vi "OutputBitAssignments.vi"(0 "System":u16(ring) items=["Cusp", "Positron", "Musashi"]) -> ()   [LabVIEW 2018]
panel:
  in  "Close (enter)":bool
  out "message":string="Output Bit Assignments\n-------------------------\n00 DAQ trigger\n01 \n02 Sync accumulator\n03 MCP select\n04 MCP in\n05 MCP out\n06 e- source select\n07 e- source insert\n08 e- source remove\n09 e- source pulse\n10 u5 AC bypass relay\n11 u10 AC bypass relay\n12 u13 AC bypass relay"
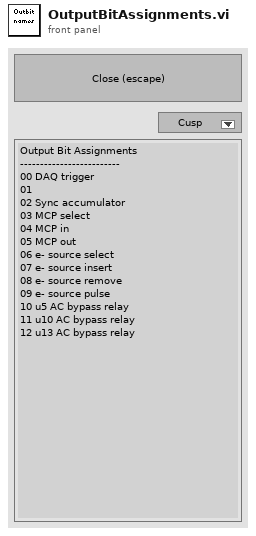
[diagram p1: front panel]
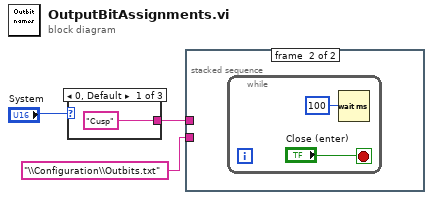
[diagram p0: block diagram]
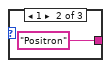
[diagram p2: hidden frame]
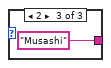
[diagram p3: hidden frame]
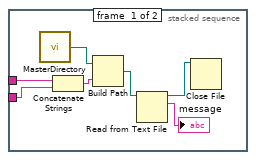
[diagram p4: hidden frame]
diagram:
  n1 = case shown="0, Default" "System" {
    tunnel: ["Cusp" ("string") "Positron" ("string") "Musashi" ("string")] -> w2
    frame 0, Default {
    }
    frame 1 {
    }
    frame 2 {
    }
  }
  n2 = stacked-sequence {
    tunnel: w2 -> [w12 _]
    tunnel: "\\Configuration\\Outbits.txt" ("string") -> [w8 _]
    frame #0 {
      n3 = call "MasterDirectory.vi"() -> ("Master Directory"=w11:path)
      n4 = Concatenate Strings(w12, w8) -> (w10:string)
      n5 = Build Path(base path=w11, name or relative path=w10) -> (appended path=w9:path)
      n6 = Read from Text File(file (use dialog)=w9) -> (refnum out=w13:refnum<file>, text=→"message":string)  [unwired: 3 in, 2 out]
      n7 = Close File(refnum=w13) -> ()  [unwired: 1 in, 2 out]
    }
    frame #1 {
      n8 = while {
        stop <- "Close (enter)" stop-if-true
        n9 = Wait (ms)(milliseconds to wait=u32 100) -> ()  [unwired: 1 out]
      }
    }
  }
